vi "RSZVB Getting Started.vi"() -> ()   [LabVIEW 2011]
doc: "This VI is an simple example how to use instrument driver VIs."
panel:
  in  "Start Frequency (300.0e3 Hz)":dbl=300000.0 format="%^.3e"
  in  "Stop Frequency (4.0e9 Hz)":dbl=4000000000.0 format="%^.3e"
  in  "Power (0.0 dBm)":dbl format="%^.3e"
  out "Measurement Status":string
  out "error out":errorcluster {"code" format="%.0x"}
  out "XY Graph":cluster{"Trace Data":dbl[], "Trace Data":dbl[]}(graph)={"Trace Data"=[300000.0, 20298500.0, 40297000.0, 60295500.0, 80294000.0, 100292496.0, 120291000.0, 140289504.0, 160288000.0, 180286496.0, 200284992.0, 220283504.0, 240282000.0, 260280496.0, 280279008.0, 300277504.0, 320276000.0, 340274496.0, 360272992.0, 380271488.0, 400270016.0, 420268512.0, 440267008.0, 460265504.0, 480264000.0, 500262496.0, 520260992.0, 540259520.0, 560257984.0, 580256512.0, 600254976.0, 620253504.0, 640252032.0, 660250496.0, 680249024.0, 700247488.0, 720246016.0, 740244480.0, 760243008.0, 780241472.0, 800240000.0, 820238528.0, 840236992.0, 860235520.0, 880233984.0, 900232512.0, 920230976.0, 940229504.0, 960227968.0, 980226496.0, 1000225024.0, 1020223488.0, 1040222016.0, 1060220480.0, 1080219008.0, 1100217472.0, 1120216064.0, 1140214528.0, 1160212992.0, 1180211456.0, 1200210048.0, 1220208512.0, 1240206976.0, 1260205440.0, 1280204032.0, 1300202496.0, 1320200960.0, 1340199552.0, 1360198016.0, 1380196480.0, 1400194944.0, 1420193536.0, 1440192000.0, 1460190464.0, 1480189056.0, 1500187520.0, 1520185984.0, 1540184448.0, 1560183040.0, 1580181504.0, 1600179968.0, 1620178560.0, 1640177024.0, 1660175488.0, 1680173952.0, 1700172544.0, 1720171008.0, 1740169472.0, 1760167936.0, 1780166528.0, 1800164992.0, 1820163456.0, 1840162048.0, 1860160512.0, 1880158976.0, 1900157440.0, 1920156032.0, 1940154496.0, 1960152960.0, 1980151552.0, 2000150016.0, 2020148480.0, 2040146944.0, 2060145536.0, 2080144000.0, 2100142464.0, 2120141056.0, 2140139520.0, 2160137984.0, 2180136448.0, 2200134912.0, 2220133376.0, 2240132096.0, 2260130560.0, 2280129024.0, 2300127488.0, 2320125952.0, 2340124416.0, 2360122880.0, 2380121600.0, 2400120064.0, 2420118528.0, 2440116992.0, 2460115456.0, 2480113920.0, 2500112384.0, 2520111104.0, 2540109568.0, 2560108032.0, 2580106496.0, 2600104960.0, 2620103424.0, 2640101888.0, 2660100608.0, 2680099072.0, 2700097536.0, 2720096000.0, 2740094464.0, 2760092928.0, 2780091392.0, 2800090112.0, 2820088576.0, 2840087040.0, 2860085504.0, 2880083968.0, 2900082432.0, 2920080896.0, 2940079616.0, 2960078080.0, 2980076544.0, 3000075008.0, 3020073472.0, 3040071936.0, 3060070400.0, 3080069120.0, 3100067584.0, 3120066048.0, 3140064512.0, 3160062976.0, 3180061440.0, 3200059904.0, 3220058624.0, 3240057088.0, 3260055552.0, 3280054016.0, 3300052480.0, 3320050944.0, 3340049408.0, 3360048128.0, 3380046592.0, 3400045056.0, 3420043520.0, 3440041984.0, 3460040448.0, 3480038912.0, 3500037376.0, 3520036096.0, 3540034560.0, 3560033024.0, 3580031488.0, 3600029952.0, 3620028416.0, 3640026880.0, 3660025600.0, 3680024064.0, 3700022528.0, 3720020992.0, 3740019456.0, 3760017920.0, 3780016384.0, 3800015104.0, 3820013568.0, 3840012032.0, 3860010496.0, 3880008960.0, 3900007424.0, 3920005888.0, 3940004608.0, 3960003072.0, 3980001536.0, 4000000000.0], "Trace Data"=[-60.757598876953125, -81.51158142089844, -76.36953735351562, -75.75534057617188, -90.45052337646484, -94.71012115478516, -88.98258209228516, -83.97650909423828, -80.61318969726562, -87.21561431884766, -87.58088684082031, -84.27996826171875, -83.89330291748047, -86.85409545898438, -95.49897003173828, -91.78004455566406, -92.24752044677734, -91.49402618408203, -86.00450134277344, -88.43099975585938, -85.20719146728516, -99.04955291748047, -95.28717803955078, -84.83718872070312, -85.83609771728516, -80.2082290649414, -92.79255676269531, -97.8532943725586, -93.57888793945312, -91.43961334228516, -82.26358032226562, -86.8819580078125, -90.0052719116211, -80.06473541259766, -80.95722961425781, -86.09173583984375, -88.3076171875, -90.39221954345703, -87.71260833740234, -96.396728515625, -91.20486450195312, -93.14900207519531, -87.56864166259766, -93.01896667480469, -87.15876007080078, -91.87611389160156, -96.0020751953125, -90.20059967041016, -86.23272705078125, -90.2487564086914, -94.52925872802734, -90.083740234375, -88.71176147460938, -85.34606170654297, -88.14515686035156, -90.61959075927734, -86.30850219726562, -82.83778381347656, -98.11040496826172, -93.22175598144531, -95.79312133789062, -89.74114227294922, -86.77118682861328, -85.09503936767578, -98.4458999633789, -108.06163024902344, -87.37747955322266, -81.79789733886719, -91.49616241455078, -90.54225158691406, -88.21485137939453, -89.33564758300781, -98.0006332397461, -93.17096710205078, -94.83616638183594, -89.43790435791016, -88.86183166503906, -85.6646728515625, -93.98345947265625, -98.86397552490234, -100.8582534790039, -87.20945739746094, -87.38671112060547, -84.4298324584961, -93.33087921142578, -92.70307159423828, -83.13152313232422, -86.54978942871094, -97.07479858398438, -87.90235900878906, -86.79354858398438, -92.5835189819336, -89.22515106201172, -85.8564453125, -85.48161315917969, -92.77310943603516, -83.24888610839844, -95.56130981445312, -87.79869079589844, -80.08671569824219, -89.0944595336914, -95.19857788085938, -107.70245361328125, -88.8790512084961, -95.084716796875, -94.32196807861328, -89.42558288574219, -96.79866790771484, -89.0506820678711, -93.91204071044922, -86.02366638183594, -89.52008819580078, -88.63750457763672, -93.82249450683594, -98.63877868652344, -90.68707275390625, -88.37232971191406, -101.31080627441406, -84.6117935180664, -89.70203399658203, -107.9026870727539, -91.02275848388672, -93.31209564208984, -90.14833068847656, -87.99365997314453, -83.4564437866211, -87.27273559570312, -88.35212707519531, -85.28385162353516, -82.47013092041016, -84.9009017944336, -82.74092102050781, -89.950927734375, -90.0771255493164, -94.65461730957031, -82.989501953125, -94.6248779296875, -86.37838745117188, -84.56217193603516, -91.93521881103516, -81.98065185546875, -87.89429473876953, -96.11864471435547, -100.66309356689453, -85.84132385253906, -86.56464385986328, -93.16865539550781, -88.483154296875, -86.92390441894531, -84.78076171875, -92.4830551147461, -90.91521453857422, -91.74028015136719, -93.38834381103516, -87.7472152709961, -86.92694854736328, -91.26090240478516, -91.21998596191406, -81.7416763305664, -95.28966522216797, -95.0335922241211, -102.62908935546875, -86.23252868652344, -94.85983276367188, -92.16241455078125, -100.17193603515625, -91.1637954711914, -83.97006225585938, -87.425048828125, -82.96971893310547, -113.03657531738281, -90.5382080078125, -105.69107055664062, -101.34162139892578, -87.37138366699219, -92.19261169433594, -89.83759307861328, -105.74420166015625, -82.63597869873047, -88.75691986083984, -85.76876068115234, -82.84273529052734, -89.49774169921875, -82.23396301269531, -87.79834747314453, -89.0394515991211, -89.35384368896484, -80.47793579101562, -81.29552459716797, -93.65138244628906, -88.41831970214844, -97.466064453125, -95.74734497070312, -82.0538101196289, -89.07303619384766, -94.23091888427734, -83.53889465332031, -95.55655670166016, -88.4918441772461, -81.2625961303711, -84.49398803710938]}
  in  "ID Query?":bool=TRUE
  in  "Reset?":bool=TRUE
  in  "VISA Resource Name":refnum<visa-resource-name>
  # "Rohde&Schwarz ZVB Network Analyzer"
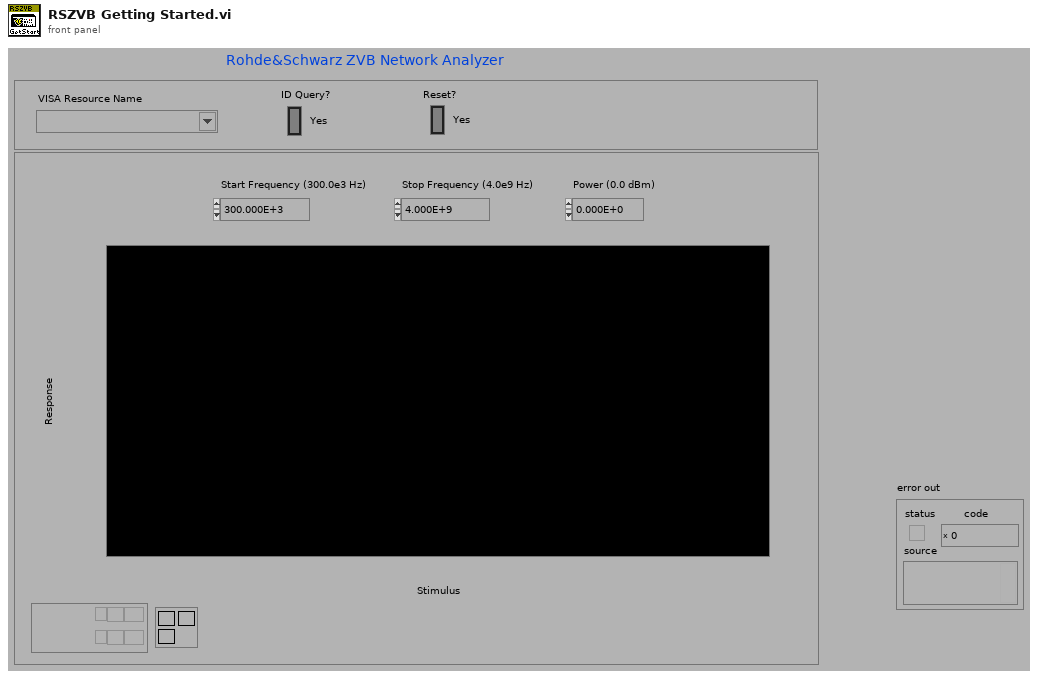
[diagram p1: front panel]
types:
  T1 = cluster{"Stimulus Data":dbl[], "Response Data":dbl[]}
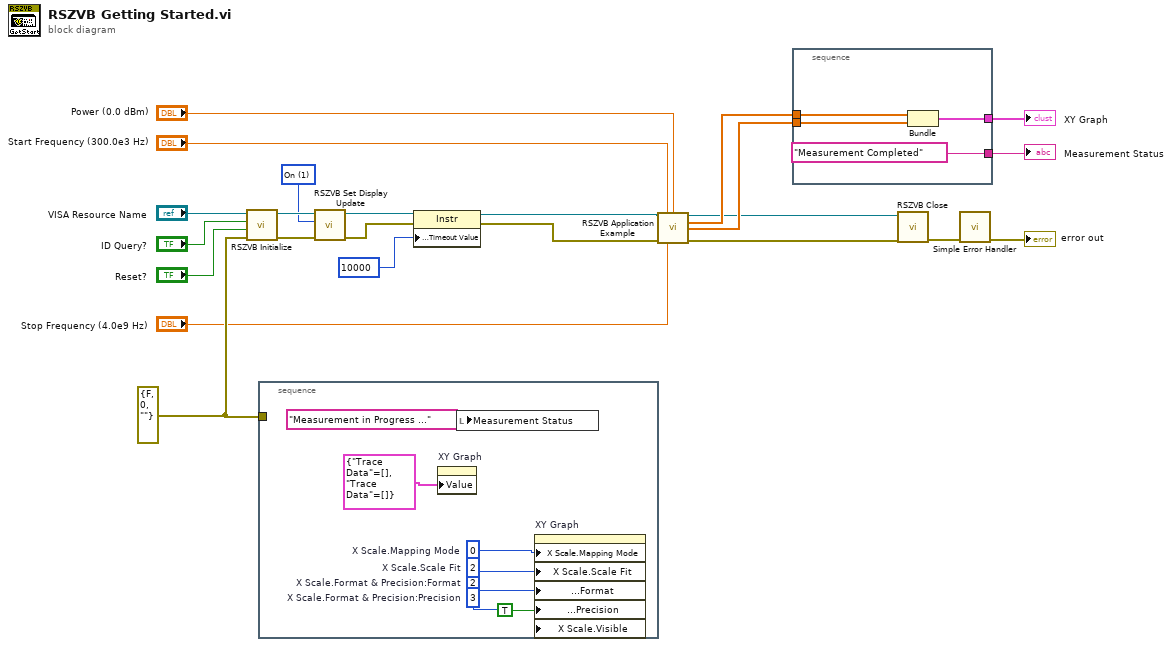
[diagram p0: block diagram]
diagram:
  w13 = 1 items=["Off", "On", "Once"] ("Display Update (0: Off)")
  w4 = errorcluster {"status"=FALSE, "code"=0, "source"=""} ("error in (no error)")
  n1 = call "RSZVB Initialize.vi"("error in (no error)"=w4, "Reset? (T: Yes)"="Reset?", "ID Query? (T: Yes)"="ID Query?", "VISA Resource Name (GPIB::20)"="VISA Resource Name") -> ("error out"=w19:errorcluster, "dup VISA session"=w20:refnum<visa-resource-name>)  [unwired: 6 in]
  n2 = stacked-sequence {
    tunnel: w4 -> [_]
    frame #0 {
      w25 = u8 0  # X Scale.Mapping Mode
      w27 = u8 2  # X Scale.Format & Precision:Format
      w28 = u8 3  # X Scale.Format & Precision:Precision
      w26 = u8 2  # X Scale.Scale Fit
      n3 = property on="XY Graph" class="XYGraph (strict)"("Value"=cluster{"Trace Data":dbl[], "Trace Data":dbl[]} {"Trace Data"=[], "Trace Data"=[]} ("XY Graph")) -> ()  [unwired: 2 in, 2 out]
      n4 = local write "Measurement Status"("Measurement in Progress ...") -> ()
      n5 = property on="XY Graph" class="XYGraph (strict)"("X Scale.Mapping Mode"=w25, "X Scale.Scale Fit"=w26, "X Scale.Format & Precision:Format"=w27, "X Scale.Format & Precision:Precision"=w28, "X Scale.Visible"=TRUE) -> ()  [unwired: 2 in, 2 out]
    }
  }
  n6 = call "RSZVB Set Display Update.vi"("error in (no error)"=w19, "Display Update (0: Off)"=w13, "VISA session"=w20) -> ("error out"=w17:errorcluster, "dup VISA session"=w18:refnum<visa-resource-name>)  [unwired: 7 in]
  n7 = property class="Instr"(reference=w18, error in=w17, "General Settings:Timeout Value"=u32 10000) -> (reference out=w11:refnum<visa-resource-name>, error out=w10:errorcluster)
  n8 = call "RSZVB Application Example.vi"("VISA session"=w11, "Start Frequency (300.0e3 Hz)"="Start Frequency (300.0e3 Hz)", "Power (0.0 dBm)"="Power (0.0 dBm)", "error in (no error)"=w10, "Stop Frequency (4.0e9 Hz)"="Stop Frequency (4.0e9 Hz)") -> ("dup VISA session"=w7:refnum<visa-resource-name>, "Stimulus Data"=w9:dbl[], "Response Data"=w8:dbl[], "error out"=w6:errorcluster)  [unwired: 7 in]
  n9 = stacked-sequence {
    tunnel: [w34] -> w5
    tunnel: ["Measurement Completed"] -> w12
    tunnel: w9 -> [w32]
    tunnel: w8 -> [w31]
    frame #0 {
      n10 = Bundle("Stimulus Data"=w32, "Response Data"=w31) -> (w34:T1)  [unwired: 1 in]
    }
  }
  "Measurement Status" <- w12
  "XY Graph" <- w5
  n11 = call "RSZVB Close.vi"("error in (no error)"=w6, "VISA session"=w7) -> ("error out"=w15:errorcluster)  [unwired: 9 in]
  n12 = call <vilib>:"Simple Error Handler.vi"("error in (no error)"=w15) -> ("error out"=→"error out":errorcluster)  [unwired: 4 in, 4 out]
